vi "Test-api.vi"() -> ()   [LabVIEW 2017, in "tmpevent.lvlib"]
uses:
  tmpevent.lvlib
  Communication/Communication.lvlib
panel:
  out "error out":errorcluster
  out "Response":variant
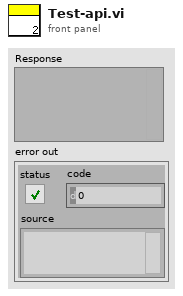
[diagram p1: front panel]
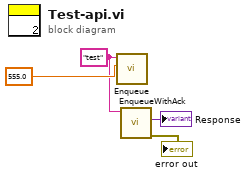
[diagram p0: block diagram]
diagram:
  w3 = "test" ("Msg")
  n1 = call "Enqueue.vi"("Data"=555.0, "Msg"=w3) -> ()  [unwired: 9 in, 1 out]
  n2 = call "EnqueueWithAck.vi"("Msg"=w3) -> ("error out"=→"error out":errorcluster, "Response"=→"Response":variant)  [unwired: 9 in]
